vi "frequencysignals.vi"() -> ()   [LabVIEW 2015]
panel:
  out "Sine":dynamicdata(graph)
  in  "Fase(°)":dbl(knob) scale=0.0..10.0
  in  "Offset (V)":dbl(knob) scale=0.0..10.0
  in  "Frecuencia (Hz)":dbl(knob) scale=0.0..500.0
  in  "Amplitud (V)":dbl(knob) scale=0.0..10.0
  in  "stop":bool
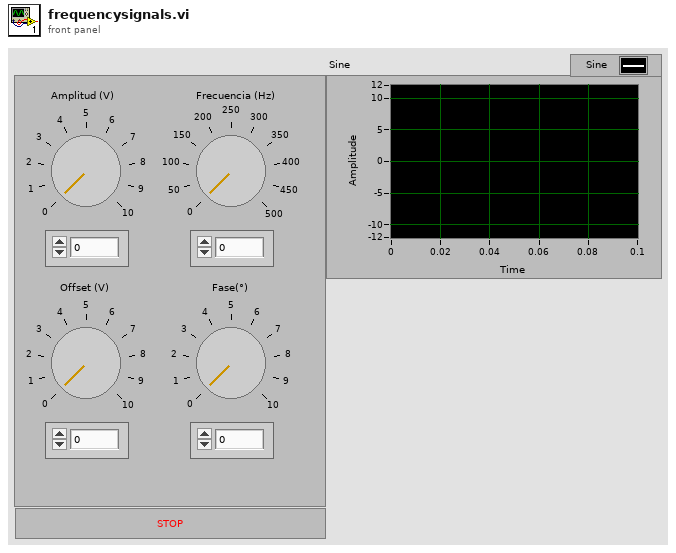
[diagram p1: front panel]
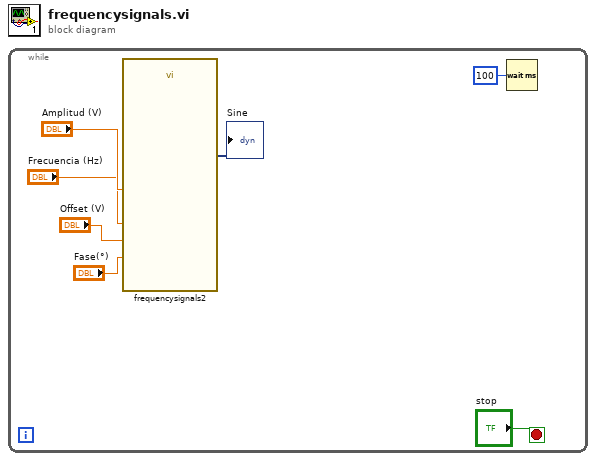
[diagram p0: block diagram]
diagram:
  n1 = while {
    stop <- "stop" stop-if-true
    n2 = call "frequencysignals2.vi"("Offset"="Offset (V)", "Frequency"="Frecuencia (Hz)", "Amplitude"="Amplitud (V)", "Phase"="Fase(°)") -> ("Sine"=→"Sine":dynamicdata)  [unwired: 10 in, 1 out]
    n3 = Wait (ms)(milliseconds to wait=u32 100) -> ()  [unwired: 1 out]
  }
